vi "RN_Motor_Einschalten.vi"(6 "error in":errorcluster, 8 "Motorwahl":string(combo)="0", 9 "VISA resource name in":refnum<visa-resource-name>) -> (0 "error out":errorcluster, 1 "Motor eingeschaltet [True]":bool=TRUE, 2 "Gesendeter Code":string, 3 "VISA resource name out":refnum<visa-resource-name>)   [LabVIEW 2014]
doc: "VI zum Einschalten der Motoren der RN-Motorsteuerung;"
panel:
  in  "Steuercode":string="o"
  in  "Kennung - RN-Motorsteuerung":string="#rm"
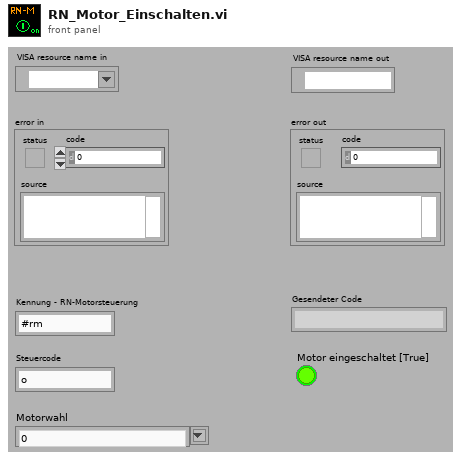
[diagram p1: front panel]
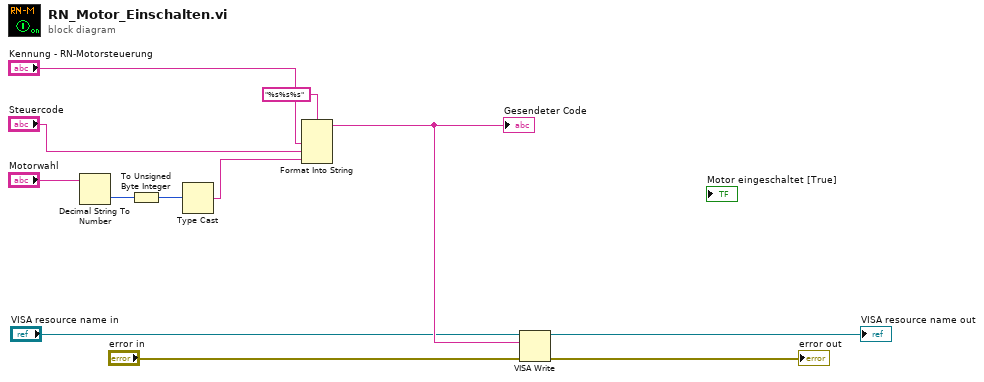
[diagram p0: block diagram]
diagram:
  n1 = Decimal String To Number(string="Motorwahl") -> (number=w11:i32)  [unwired: 2 in, 1 out]
  n2 = To Unsigned Byte Integer(number=w11) -> (unsigned 8bit integer=w10:u8)
  n3 = Type Cast(x=w10) -> (*(type *) &x=w7:string)  [unwired: 1 in]
  n4 = Format Into String(format string="%s%s%s", "Kennung - RN-Motorsteuerung", "Steuercode", w7) -> (resulting string=w5:string)  [unwired: 2 in, 1 out]
  "Gesendeter Code" <- w5
  n5 = VISA Write(VISA resource name="VISA resource name in", write buffer=w5, error in (no error)="error in") -> (VISA resource name out=→"VISA resource name out":refnum<visa-resource-name>, error out=→"error out":errorcluster)  [unwired: 1 out]
